vi "pyWebscraper.vi"(7 "pyWebscraper Test Type":T2, 8 "error in (no error)":errorcluster, 9 "Image Configuration":T1={"Images"=[], "Confidence"=0.9} caption="Image Configuration (Only applicable for ratio test)" {"Confidence" min=0.0 max=1.0 format="%.2g"}, 10 "pyWebscraper Configuration":T3={"URL"="", "Delay (s)"=10} {"Delay (s)" max=1}, 11 "Python Directory":path caption="(Example: C:\\Program Files\\SEGGER\\JLink)") -> (0 "error out":errorcluster, 1 "PASS":bool, 2 "2D Array":string[][](array[string]), 3 "Output":string)   [LabVIEW 2016, in "Webscraper.lvlib"]
doc: "This VI performs Flash Programming through JLink Commander."
uses:
  Webscraper.lvlib
  Type Definitions/pyWebscraper Configuration.ctl
  Type Definitions/pyWebscraper Test Type.ctl
  Type Definitions/pyWebscraper Image Configuration.ctl
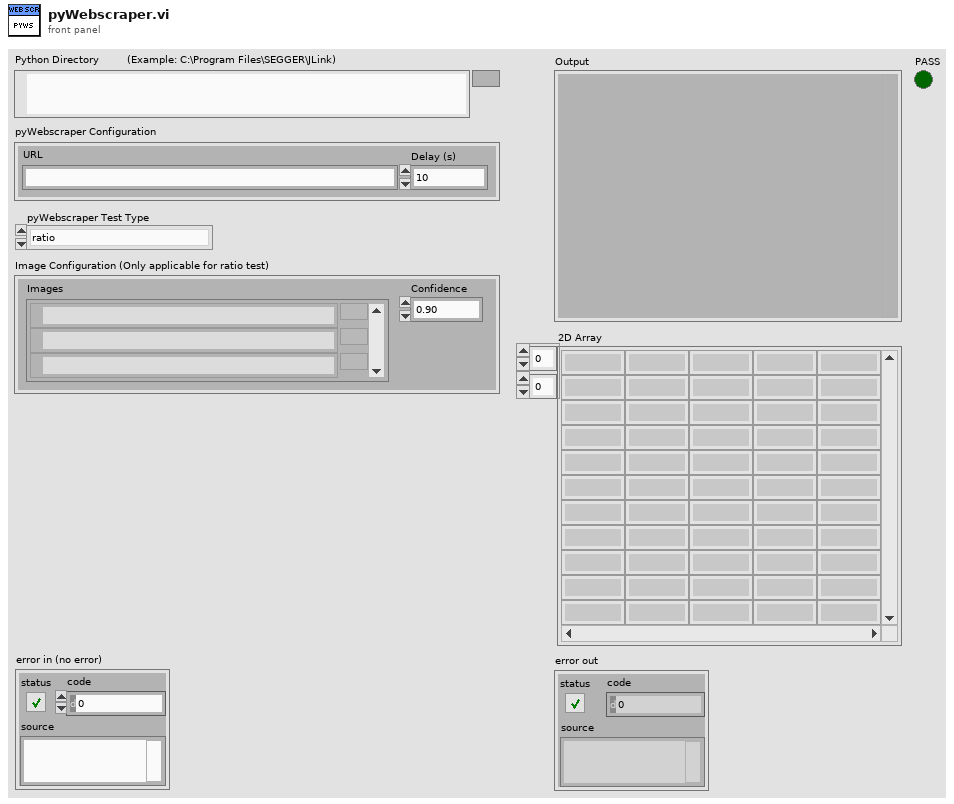
[diagram p1: front panel]
types:
  T1 = typedef "Webscraper.lvlib/pyWebscraper Image Configuration.ctl" = cluster{"Images":path[], "Confidence":dbl}
  T2 = typedef "Webscraper.lvlib/pyWebscraper Test Type.ctl" = enum16{"ratio", "overview", "livepara", "counts", "maxvalue", "alarm_ph2", "nwconfig"}
  T3 = typedef "Webscraper.lvlib/pyWebscraper Configuration.ctl" = cluster{"URL":string, "Delay (s)":u32}
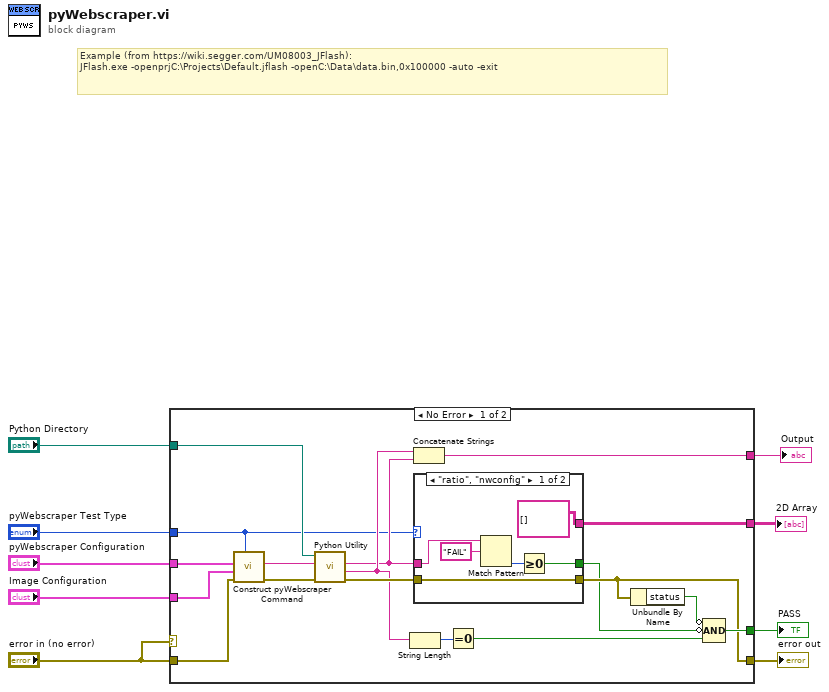
[diagram p0: block diagram]
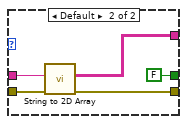
[diagram p2: hidden frame]
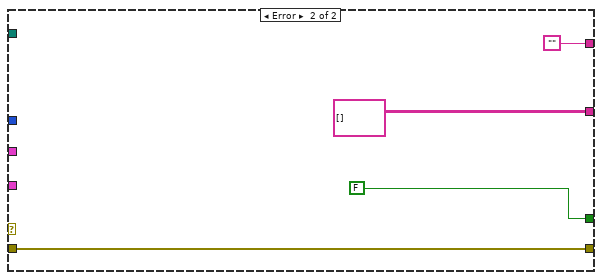
[diagram p3: hidden frame]
diagram:
  # "Example (from https://wiki.segger.com/UM08003_JFlash):\nJFlash.exe -openprjC:\\Projects\\Default.jflash -openC:\\Data\\data.bin,0x100000 -auto -exit"
  n1 = case shown="No Error" "error in (no error)" {
    tunnel: [w12 w39] -> w9
    tunnel: "Python Directory" -> [w27 _]
    tunnel: [w16 ""] -> w8
    tunnel: [w14 FALSE] -> w6
    tunnel: "pyWebscraper Configuration" -> [w25 _]
    tunnel: [w23 string[][] [] ("2D Array")] -> w4
    tunnel: "pyWebscraper Test Type" -> [w15 _]
    tunnel: "Image Configuration" -> [w22 _]
    tunnel: "error in (no error)" -> [w17 w39]
    frame No Error {
      n2 = call "Construct pyWebscraper Command.vi"("pyWebscraper Test Type"=w15, "error in (no error)"=w17, "Image Configuration"=w22, "pyWebscraper Configuration"=w25) -> ("error out"=w21:errorcluster, "pyWebscraper Command"=w26:string)  [unwired: 6 in]
      n3 = call "Python Utility.vi"("error in (no error)"=w21, "Parameters String"=w26, "Python Directory"=w27) -> ("error out"=w20:errorcluster, "standard error"=w19:string, "standard output"=w18:string)  [unwired: 6 in]
      n4 = String Length(string=w19) -> (length=w24:i32)
      n5 = Concatenate Strings(w19, w18) -> (w16:string)
      n6 = case shown="\"ratio\", \"nwconfig\"" w15 {
        tunnel: [string[][] [] ("2D Array") w38] -> w23
        tunnel: w20 -> [w32 w37]
        tunnel: w18 -> [w31 w36]
        tunnel: [w32 w35] -> w12
        tunnel: [w28 FALSE] -> w10
        frame "ratio", "nwconfig" {
          n7 = Match Pattern(string=w31, regular expression="FAIL") -> (offset past match=w29:i32)  [unwired: 1 in, 3 out]
          n8 = Greater Or Equal To 0?(x=w29) -> (x >= 0?=w28:bool)
        }
        frame Default {
          n9 = call "String to 2D Array.vi"("error in (no error)"=w37, "String"=w36) -> ("error out"=w35:errorcluster, "2D Array"=w38:string[][])  [unwired: 8 in]
        }
      }
      n10 = Equal To 0?(x=w24) -> (x = 0?=w13:bool)
      n11 = Unbundle By Name(w12) -> ("status"=w11:bool)
      n12 = Compound Arithmetic op=AND(invert w11, invert w10, w13) -> (w14:bool)
    }
    frame Error {
    }
  }
  "error out" <- w9
  "Output" <- w8
  "PASS" <- w6
  "2D Array" <- w4
